vi "xps_panel_handle_error.vi"(8 "error in (no error)":errorcluster, 11 "newport_xps_panel in":refnum<class "newport_xps_panel.lvclass">) -> (0 "error out":errorcluster, 3 "newport_xps_panel out":refnum<class "newport_xps_panel.lvclass">)   [LabVIEW 2015, in "newport_xps_panel.lvclass"]
uses:
  newport_xps_panel.lvclass
  newport_xps_panel.lvclass/newport_xps_panel.ctl
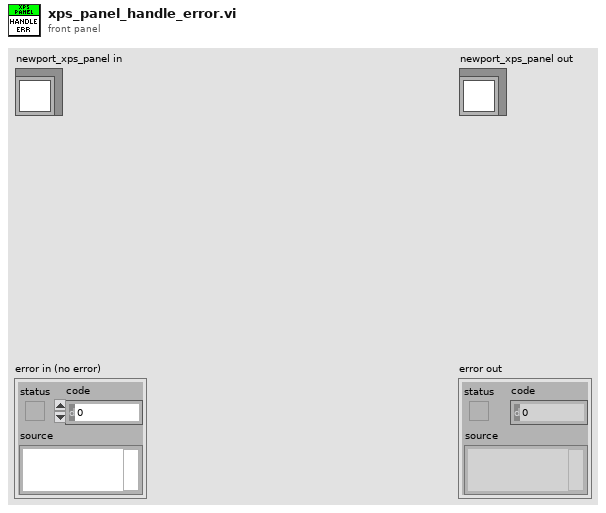
[diagram p1: front panel]
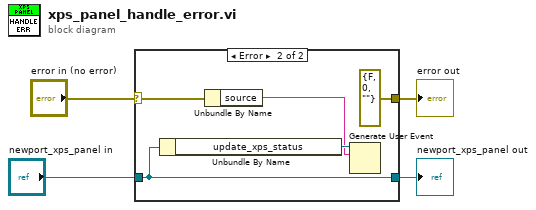
[diagram p0: block diagram]
diagram:
  n1 = case shown="Error" "error in (no error)" {
    selector: "error in (no error)" -> [w5 w10]
    tunnel: "newport_xps_panel in" -> [w6 w7]
    tunnel: [w6 w7] -> w2
    tunnel: [w5 errorcluster {"status"=FALSE, "code"=0, "source"=""} ("error IO")] -> w1
    frame No Error {
    }
    frame Error {
      n2 = Unbundle By Name(w7) -> ("update_xps_status"=w11:refnum<user-event>)
      n3 = Unbundle By Name(w10) -> ("source"=w9:string)
      n4 = Generate User Event(user event=w11, event data cluster=w9) -> ()  [unwired: 2 in, 2 out]
    }
  }
  "error out" <- w1
  "newport_xps_panel out" <- w2
